vi "isEqualOfDisplay.vi"(2 "error in (no error)":errorcluster caption="错误输入（无错误）", 3 "比对数据":T1, 4 "原始数据":T1) -> (0 "error out":errorcluster caption="错误输出", 1 "布尔":bool)   [LabVIEW 2019]
uses:
  ctl/Display.ctl
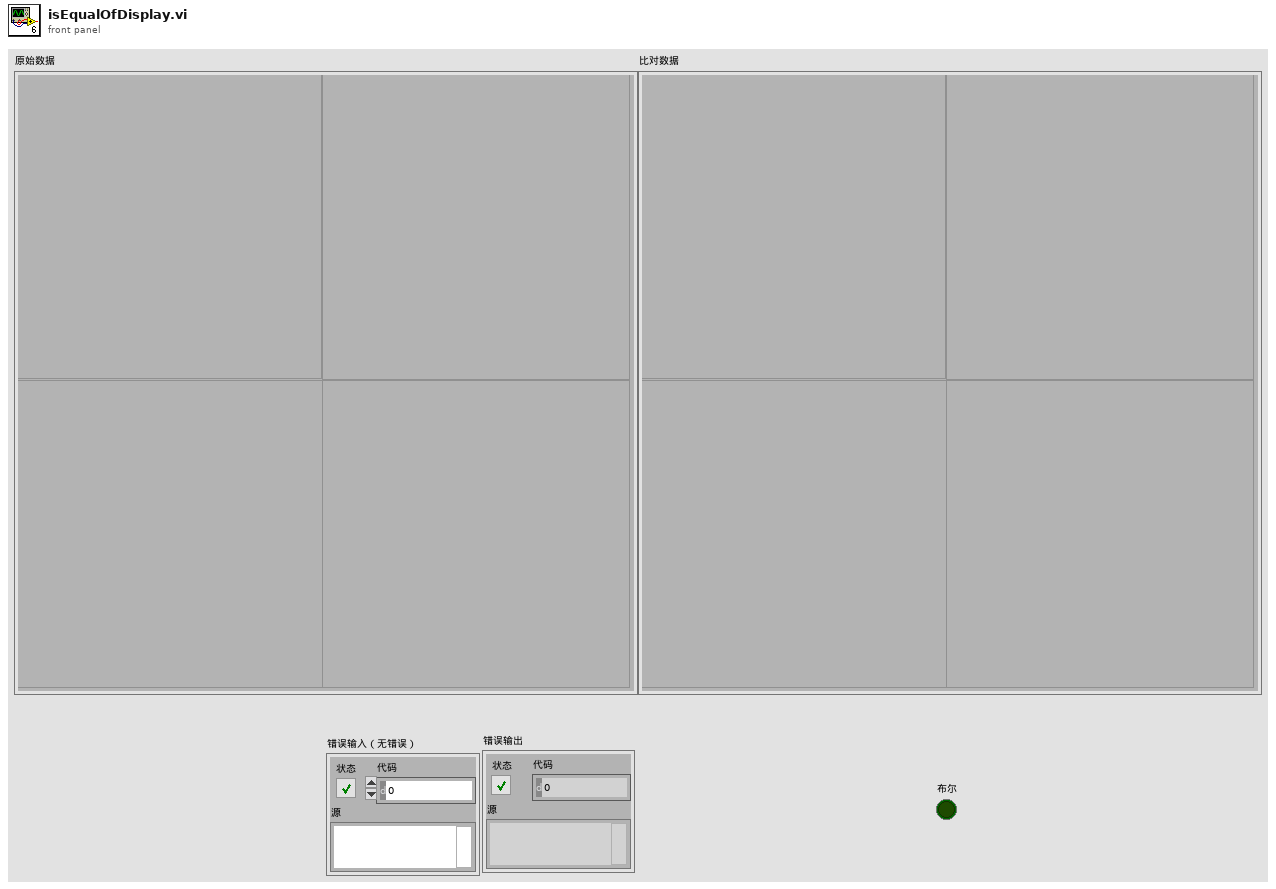
[diagram p1: front panel]
types:
  T1 = typedef "Display.ctl" = cluster{"左上":bool, "右上":bool, "左下":bool, "右下":bool}
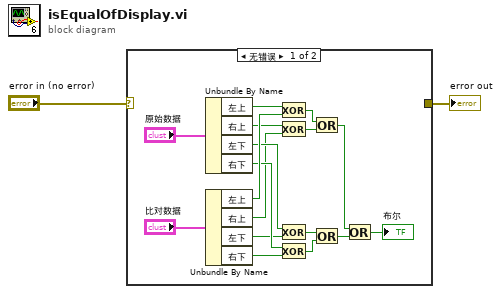
[diagram p0: block diagram]
diagram:
  n1 = case shown="无错误" "error in (no error)" {
    selector: "error in (no error)" -> [_ w20]
    tunnel: [_ w20] -> w1
    frame No Error {
      n2 = Unbundle By Name("原始数据") -> ("左上"=w17:bool, "右上"=w15:bool, "左下"=w14:bool, "右下"=w13:bool)
      n3 = Unbundle By Name("比对数据") -> ("左上"=w16:bool, "右上"=w12:bool, "左下"=w11:bool, "右下"=w10:bool)
      n4 = Exclusive Or(1:w16, 2:w17) -> (0:w9:bool)
      n5 = Exclusive Or(1:w12, 2:w15) -> (0:w8:bool)
      n6 = Exclusive Or(1:w11, 2:w14) -> (0:w7:bool)
      n7 = Exclusive Or(1:w10, 2:w13) -> (0:w6:bool)
      n8 = Or(x=w9, y=w8) -> (x .or. y?=w5:bool)
      n9 = Or(x=w7, y=w6) -> (x .or. y?=w4:bool)
      n10 = Or(x=w5, y=w4) -> (x .or. y?=→"布尔":bool)
    }
    frame Error {
    }
  }
  "error out" <- w1
